vi "ServerCommand3.vi"(0 "Command":string) -> (1 "Error":bool, 2 "Reply":string)   [LabVIEW 2014]
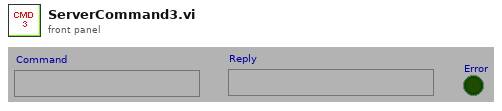
[diagram p1: front panel]
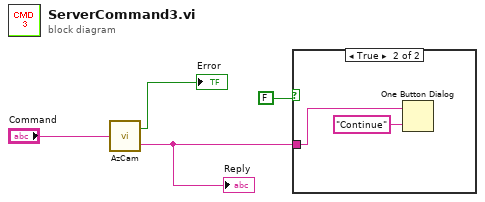
[diagram p0: block diagram]
diagram:
  n1 = call "AzCam.vi"("Command"="Command") -> ("Error"=→"Error":bool, "Reply"=w2:string)
  "Reply" <- w2
  n2 = case shown="True" FALSE {
    tunnel: w2 -> [_ w5]
    frame False {
    }
    frame True {
      n3 = One Button Dialog(message=w5, button name ("OK")="Continue") -> ()  [unwired: 1 out]
    }
  }
